vi "Close Connection.vi"(8 "error in":errorcluster, 11 "TCP slave in":refnum<class "TCP Slave.lvclass">) -> (0 "error out":errorcluster)   [LabVIEW 2012, in "TCP Slave.lvclass"]
doc: "Closes the TCP connection stored in the class."
uses:
  TCP Slave.lvclass
  TCP Slave.lvclass/TCP Slave.ctl
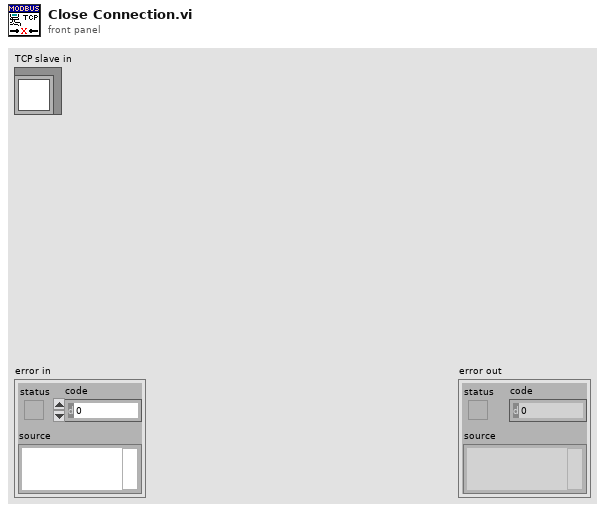
[diagram p1: front panel]
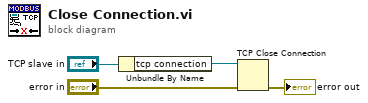
[diagram p0: block diagram]
diagram:
  n1 = Unbundle By Name("TCP slave in") -> ("tcp connection"=w3:refnum<k5>)
  n2 = TCP Close Connection(connection ID=w3, error in (no error)="error in") -> (error out=→"error out":errorcluster)  [unwired: 1 in, 1 out]
